vi "MS Updater.vi"(1 "Conveyer Belt Info":T1) -> (0 "Conveyer Belt Info out":T1)   [LabVIEW 2012]
uses:
  BotStatus.vi
panel:
  # "s"
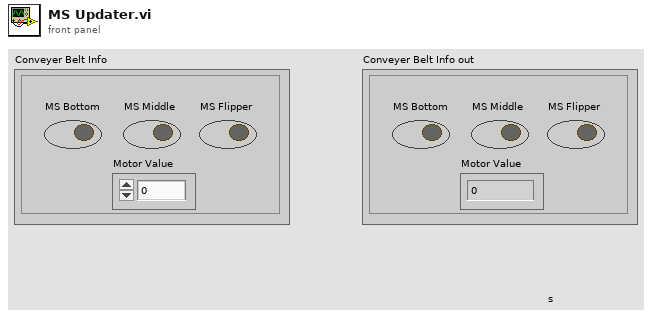
[diagram p1: front panel]
types:
  T1 = cluster{"MS Bottom":bool, "MS Middle":bool, "MS Flipper":bool, "Motor Value":dbl}
  T2 = typedef "WPI_DigitalInputDevRef.ctl" = cluster{"DevStatus":errorcluster, "DIO Channel":T3, "Digital Module":T4}
  T3 = typedef "FPGA_DIOChannel.ctl" = enum8{"DIO 1", "DIO 2", "DIO 3", "DIO 4", "DIO 5", "DIO 6", "DIO 7", "DIO 8", "DIO 9", "DIO 10", "DIO 11", "DIO 12", "DIO 13", "DIO 14", "Invalid"}
  T4 = typedef "FPGA_TypedefDigitalModule.ctl" = enum16{"Digital Module 1", "Digital Module 2"}
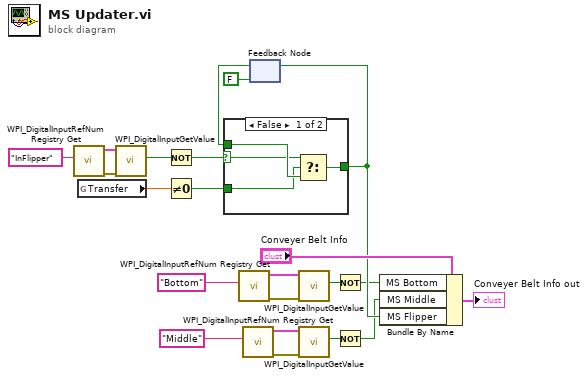
[diagram p0: block diagram]
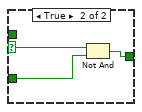
[diagram p2: hidden frame]
diagram:
  n1 = call <vilib>:"WPI_DigitalInputRefNum Registry Get.vi"("refnum name"="InFlipper") -> ("error out"=w16:errorcluster, "DigitalInputDevRef"=w15:T2)  [unwired: 9 in]
  n2 = global read "BotStatus.vi" "Transfer"() -> (w6:dbl)
  n3 = call <vilib>:"WPI_DigitalInputGetValue.vi"("error in (no error)"=w16, "DigitalInputDevRef"=w15) -> ("Value"=w10:bool)  [unwired: 7 in, 2 out]
  n4 = Not(x=w10) -> (.not. x?=w7:bool)
  n5 = Not Equal To 0?(x=w6) -> (x != 0?=w5:bool)
  n6 = call <vilib>:"WPI_DigitalInputRefNum Registry Get.vi"("refnum name"="Bottom") -> ("error out"=w17:errorcluster, "DigitalInputDevRef"=w1:T2)  [unwired: 9 in]
  n7 = call <vilib>:"WPI_DigitalInputRefNum Registry Get.vi"("refnum name"="Middle") -> ("error out"=w13:errorcluster, "DigitalInputDevRef"=w14:T2)  [unwired: 9 in]
  n8 = feedback #1(FALSE) -> (w8:bool)
  n9 = case shown="False" w7 {
    selector: w7 -> [w24 w29]
    tunnel: [w26 w28] -> w4
    tunnel: w8 -> [w25 _]
    tunnel: w5 -> [w23 w27]
    frame False {
      n10 = Select(t=w24, s=w23, f=w25) -> (s? t:f=w26:bool)
    }
    frame True {
      n11 = Not And(1:w27, 2:w29) -> (0:w28:bool)
    }
  }
  n12 = feedback-in #1(w4) -> ()
  n13 = call <vilib>:"WPI_DigitalInputGetValue.vi"("error in (no error)"=w17, "DigitalInputDevRef"=w1) -> ("Value"=w12:bool)  [unwired: 7 in, 2 out]
  n14 = call <vilib>:"WPI_DigitalInputGetValue.vi"("error in (no error)"=w13, "DigitalInputDevRef"=w14) -> ("Value"=w11:bool)  [unwired: 7 in, 2 out]
  n15 = Not(x=w12) -> (.not. x?=w2:bool)
  n16 = Not(x=w11) -> (.not. x?=w3:bool)
  n17 = Bundle By Name(cluster="Conveyer Belt Info", "MS Bottom"=w2, "MS Middle"=w3, "MS Flipper"=w4) -> (→"Conveyer Belt Info out":T1)
